vi "Insert VI.vi"(8 "error in (no error)":errorcluster, 10 "VI Ref":refnum<vi>, 11 "TestBench in":refnum<class "TestBench.lvclass">) -> (0 "error out":errorcluster, 3 "TestBench out":refnum<class "TestBench.lvclass">)   [LabVIEW 2019, in "TestBench.lvlib" / "TestBench.lvclass"]
uses:
  TestBench.lvclass
  TestBench.lvclass/TestBench.ctl
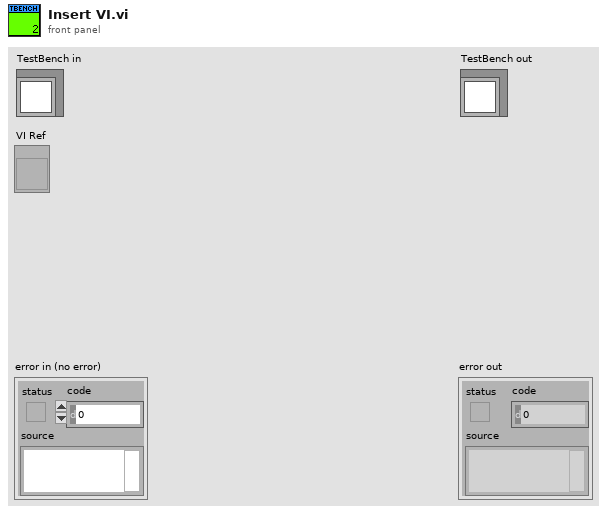
[diagram p1: front panel]
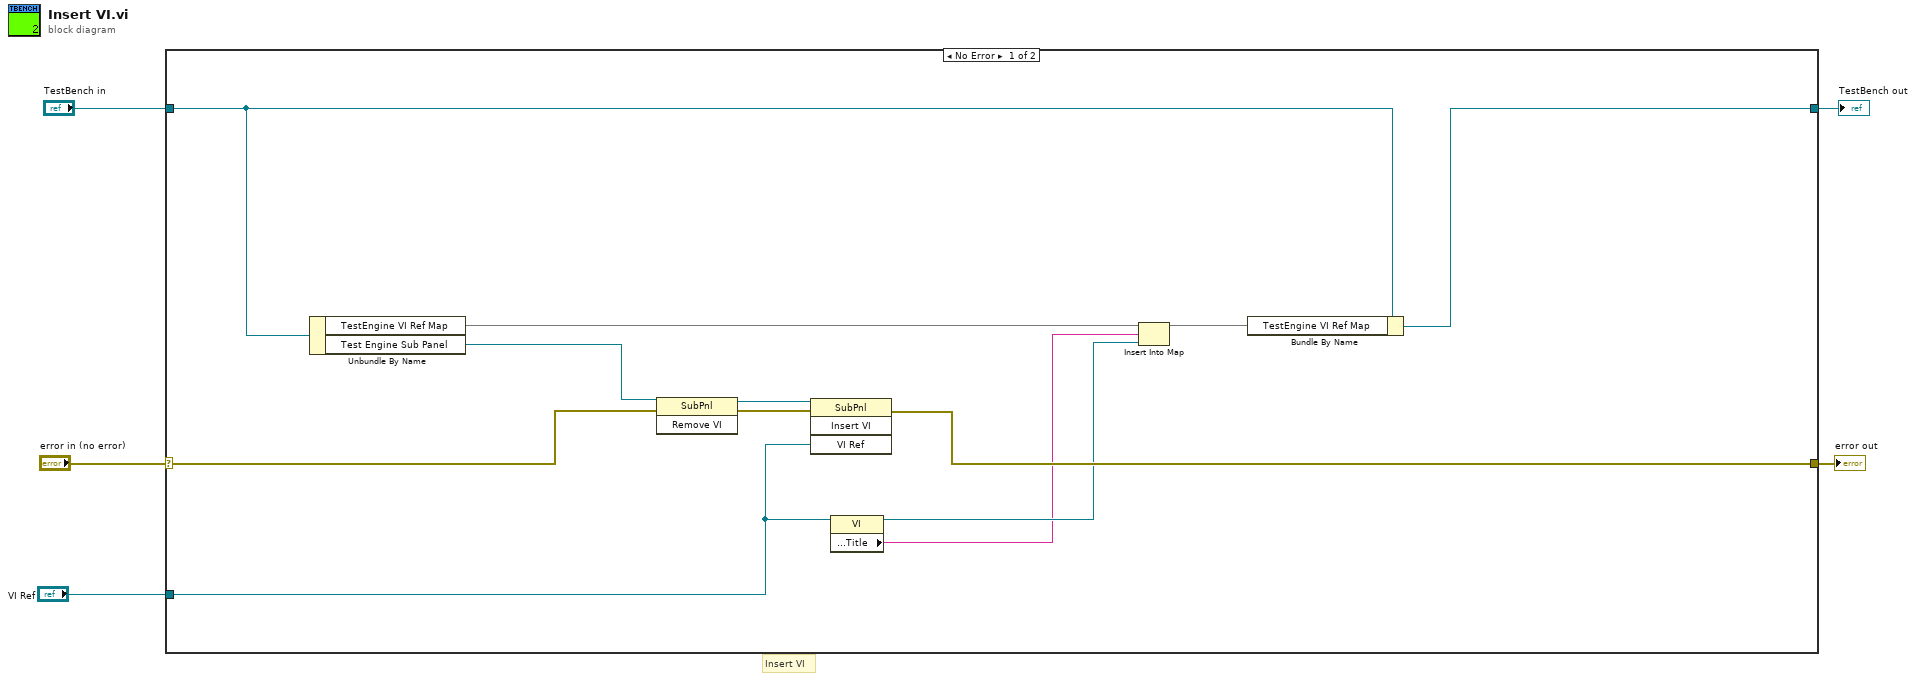
[diagram p0: block diagram]
diagram:
  # "Insert VI"
  n1 = case shown="No Error" "error in (no error)" {
    selector: "error in (no error)" -> [w17 w19]
    tunnel: [w16 w19] -> w4
    tunnel: [w13 w18] -> w2
    tunnel: "TestBench in" -> [w15 w18]
    tunnel: "VI Ref" -> [w8 _]
    frame No Error {
      n2 = Unbundle By Name(w15) -> ("TestEngine VI Ref Map"=w9:map{string, refnum<vi>}, "Test Engine Sub Panel"=w10:refnum<vi>)
      n3 = invoke class="SubPnl" method="Remove VI"(reference=w10, error in=w17) -> (reference out=w12:refnum<vi>, error out=w11:errorcluster)  [unwired: 1 in, 1 out]
      n4 = invoke class="SubPnl" method="Insert VI"(reference=w12, error in=w11, "VI Ref"=w8) -> (error out=w16:errorcluster)  [unwired: 1 in, 3 out]
      n5 = property class="VI"(reference=w8) -> (reference out=w7:refnum<vi>, "Front Panel.Title"=w6:string)  [unwired: 1 in, 1 out]
      n6 = Insert Into Map(map in=w9, key=w6, value=w7) -> (map out=w14:map{string, refnum<vi>})  [unwired: 2 out]
      n7 = Bundle By Name(cluster=w15, "TestEngine VI Ref Map"=w14) -> (w13:refnum<class "TestBench.lvclass">)
    }
    frame Error {
    }
  }
  "error out" <- w4
  "TestBench out" <- w2
